vi "readID_TCP.vi"() -> ()   [LabVIEW 2017]
panel:
  in  "long":bool=TRUE
  in  "数组 6":string[](array[string])=["shift:\u0005\u0000\u0000\u0000\u001f\u0000", "shift:\u0004\u0000\u0000\u0000\u0002\u0000", "shift: \u0000\u0000\u0000\u0000\u0000\u0000\u0000\u0000\u0000\u0000\u0000"]
  in  "数组 5":string[](array[string])=["shift: \u0000\u0000\u0000ÿÿÿÿ\u0000\u0000\u0000\u0000", "shift:(\u0000\u0000\u0000\u0002\u0000\u0000\u0000\u0000\u0000\u0000\u0000\u0000\u0000\u0000\u0000\u0000\u0000", "shift: \u0000\u0000\u0000\u0000\u0000\u0000\u0000\u0000\u0000\u0000\u0000"]
  out "k7 idcode":string
  out "sp6 idcode":string
  in  "数组 4":string[](array[string])=["settck:d\u0000\u0000\u0000"]
  in  "shift string":string="shift:\u0005\u0000\u0000\u0000\u001f\u0000"
  in  "数组 3":string[](array[string])=["shift:\u0005\u0000\u0000\u0000\u001f\u0000"]
  in  "停止":bool
  out "数值":i32=2
  out "数据输出":string
  in  "字符串 2":string="shift:\u0005\u0000\u0000\u001f\u0000"
  in  "字符串":string="getinfo:"
  in  "数组 2":string[](array[string])=["shift:\u0005\u0000\u0000\u0000\u001f\u0000", "shift:\u0004\u0000\u0000\u0000\u0002\u0000", "shift: \u0000\u0000\u0000\u0000\u0000\u0000\u0000\u0000\u0000\u0000\u0000"]
  out "错误输出":errorcluster
  in  "数组":string[](array[string])=["getinfo:"]
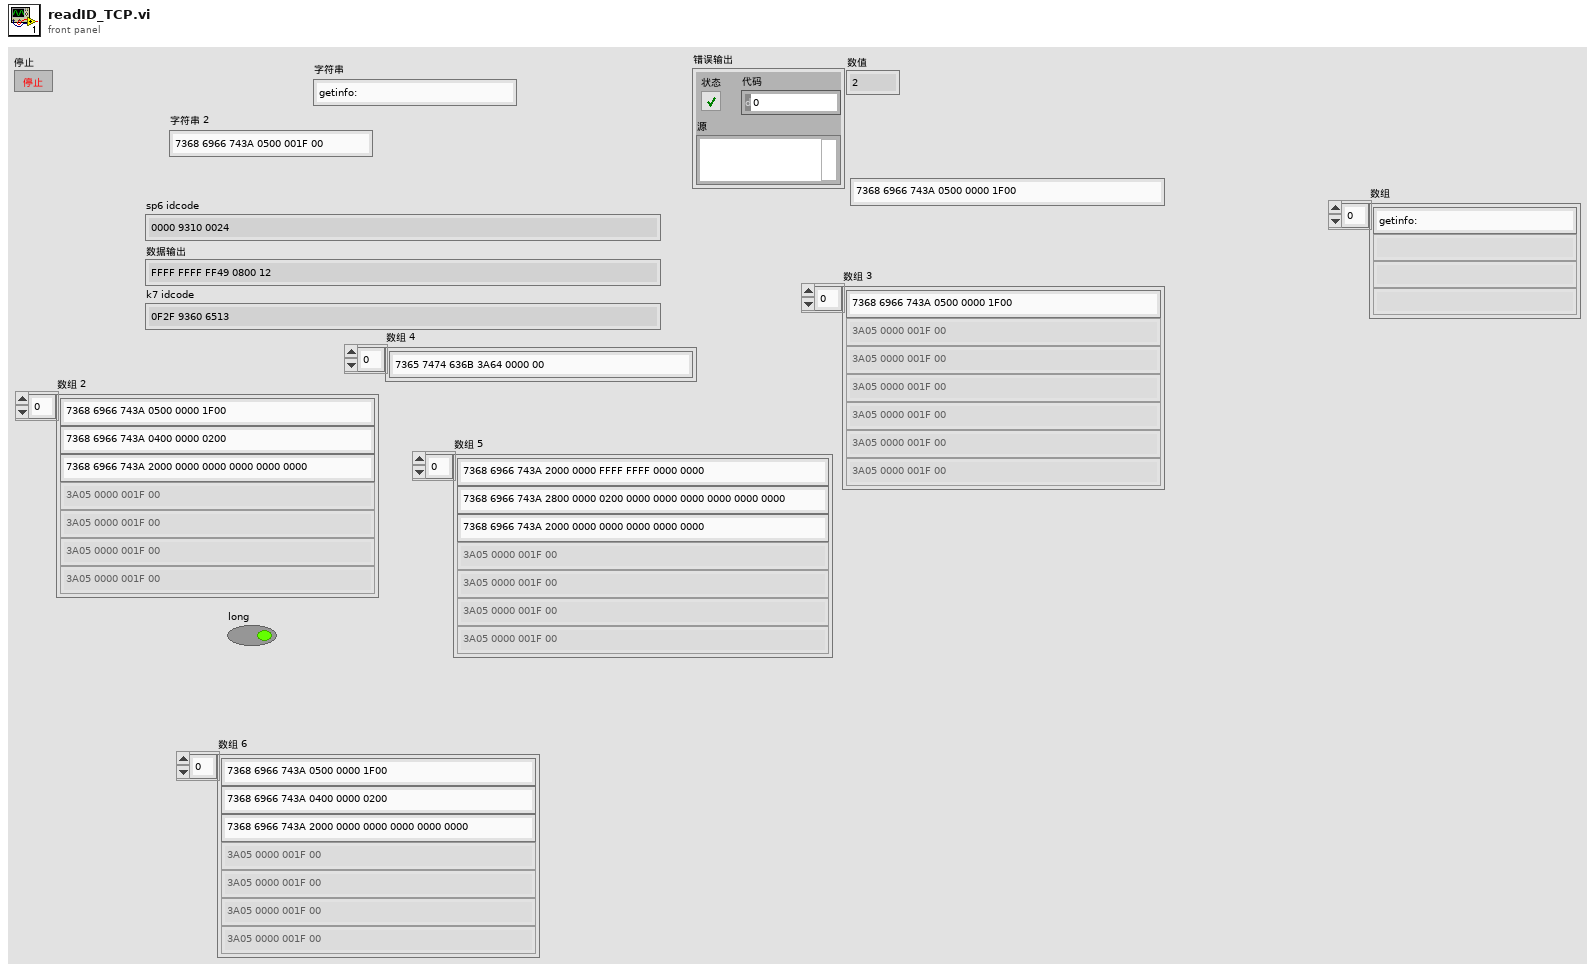
[diagram p1: front panel]
types:
  T1 = enum16{"Standard", "Buffered", "CRLF", "Immediate"}
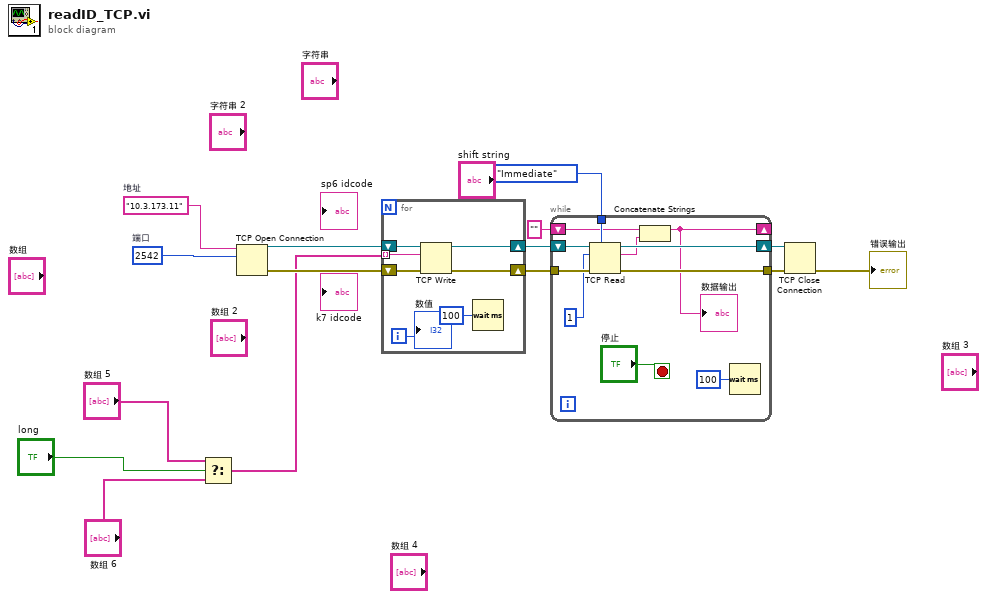
[diagram p0: block diagram]
diagram:
  w14 = u16 2542  # 端口
  w15 = "10.3.173.11"  # 地址
  n1 = Select(t="数组 5", s="long", f="数组 6") -> (s? t:f=w3:string[])
  n2 = TCP Open Connection(address=w15, remote port or service name=w14) -> (connection ID=w13:refnum<k5>, error out=w12:errorcluster)  [unwired: 3 in]
  n3 = for {
    shift-right: [w20] -> w11
    shift-left: w13 -> [w22]
    shift-right: [w19] -> w8
    shift-left: w12 -> [w21]
    tunnel: w3 -> [w18] mode=indexing
    i -> [w16]
    n4 = TCP Write(connection ID=w22, data in=w18, error in (no error)=w21) -> (connection ID out=w20:refnum<k5>, error out=w19:errorcluster)  [unwired: 1 in, 1 out]
    n5 = Wait (ms)(milliseconds to wait=u32 100) -> ()  [unwired: 1 out]
    "数值" <- w16
  }
  n6 = while {
    tunnel: T1."Immediate" ("模式（标准）") -> [w29]
    shift-right: [w32] -> w9
    shift-left: w11 -> [w33]
    shift-right: [w25] -> _
    shift-left: "" -> [w26]
    tunnel: w8 -> [w31]
    tunnel: [w30] -> w7
    stop <- "停止" stop-if-true
    n7 = TCP Read(connection ID=w33, bytes to read=1 ("读取的字节"), error in (no error)=w31, 7:w29) -> (connection ID out=w32:refnum<k5>, data out=w24:string, error out=w30:errorcluster)  [unwired: 1 in]
    n8 = Concatenate Strings(w26, w24) -> (w25:string)
    "数据输出" <- w25
    n9 = Wait (ms)(milliseconds to wait=u32 100) -> ()  [unwired: 1 out]
  }
  n10 = TCP Close Connection(connection ID=w9, error in (no error)=w7) -> (error out=→"错误输出":errorcluster)  [unwired: 1 in, 1 out]
